vi "TestTrigger.vi"() -> ()   [LabVIEW 2023, in "TDK20-38 API.lvlib"]
uses:
  TDK20-38 API.lvlib
panel:
  in  "error in (no error)":errorcluster
  in  "Device position":string
  out "error out":errorcluster
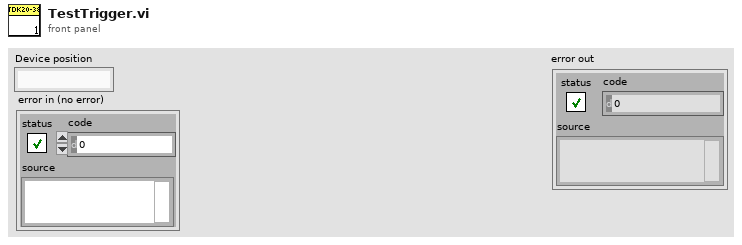
[diagram p1: front panel]
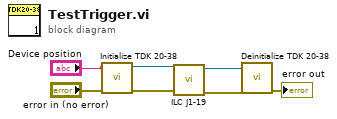
[diagram p0: block diagram]
diagram:
  n1 = call "Initialize TDK 20-38.vi"("error in (no error)"="error in (no error)", "Device position"="Device position") -> ("error out"=w3:errorcluster, "VISA out"=w7:refnum<visa-resource-name>)  [unwired: 8 in]
  n2 = call "ILC J1-19.vi"("error"=w3, "VISA"=w7) -> ("error out"=w2:errorcluster, "VISA out"=w1:refnum<visa-resource-name>)  [unwired: 8 in]
  n3 = call "Deinitialize TDK 20-38.vi"("error"=w2, "VISA name"=w1) -> ("error out"=→"error out":errorcluster)  [unwired: 9 in]
